vi "readCRC.vi"(8 "error in (no error)":errorcluster, 11 "ModbusBuffer in":refnum<class "ModbusBufferBuilder.lvclass">) -> (0 "error out":errorcluster, 2 "Output":u16, 3 "ModbusBuffer out":refnum<class "ModbusBufferBuilder.lvclass">)   [LabVIEW 2016, in "ModbusBufferBuilder.lvclass"]
uses:
  ModbusBufferBuilder.lvclass
  ModbusBufferBuilder.lvclass/ModbusBufferBuilder.ctl
  readInstructionByte.vi
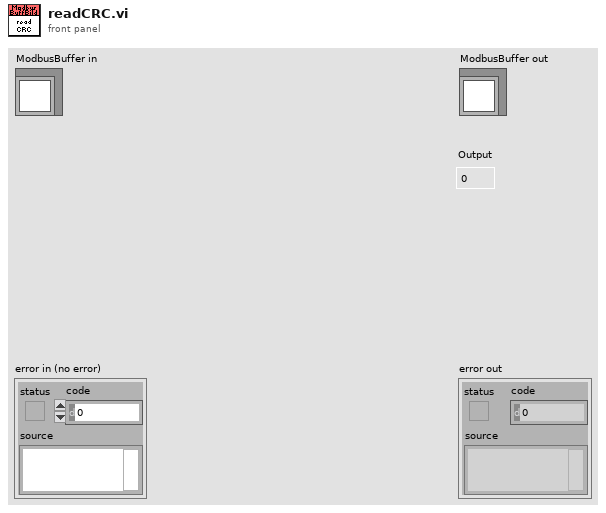
[diagram p1: front panel]
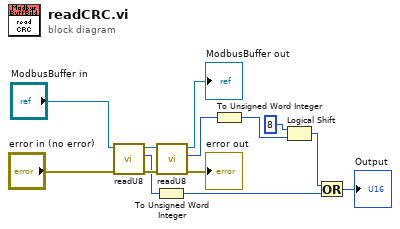
[diagram p0: block diagram]
diagram:
  n1 = call "readU8.vi"("error in (no error)"="error in (no error)", "ModbusBuffer in"="ModbusBuffer in") -> ("error out"=w5:errorcluster, "Output"=w3:u8, "ModbusBuffer out"=w11:refnum<class "ModbusBufferBuilder.lvclass">)  [unwired: 7 in]
  n2 = To Unsigned Word Integer(number=w3) -> (unsigned 16bit integer=w9:u16)
  n3 = call "readU8.vi"("error in (no error)"=w5, "ModbusBuffer in"=w11) -> ("error out"=→"error out":errorcluster, "Output"=w2:u8, "ModbusBuffer out"=→"ModbusBuffer out":refnum<class "ModbusBufferBuilder.lvclass">)  [unwired: 7 in]
  n4 = To Unsigned Word Integer(number=w2) -> (unsigned 16bit integer=w1:u16)
  n5 = Logical Shift(y=i16 8, x=w1) -> (x << y=w8:u16)
  n6 = Or(x=w8, y=w9) -> (x .or. y?=→"Output":u16)
